vi "solar_tcp Core Client.vi"(7 "Action":T4, 8 "error in (no error)":errorcluster, 9 "Read Timeout (0ms)":i32, 10 "Message to Send":string, 11 "TCP Data in":T1 {"Debug"."Time" format="%<%Y-%m-%d\n%H:%M:%S%3u>T"}) -> (0 "error out":errorcluster, 1 "Connected":bool, 2 "Message Read/Sent":string, 3 "TCP Data out":T1 {"Debug"."Time" format="%<%Y-%m-%d\n%H:%M:%S%3u>T"})   [LabVIEW 2018]
doc: "This is the TCP Client core state machine that handles a TCP session. The <b>Message to Send</b> and <b>Message Read</b> should contain the entire TCP message including the header. Before writing the <b>Message to Send</b> the length field is updated as defined by the configuration header length offset and size. The total length field is typically the first 4 bytes of the message which includes the total packet size."
uses:
  solar_tcp_ctl Action.ctl
  solar_tcp_ctl Data.ctl
  solar_tcp_ctl Config.ctl
  solar_tcp_ctl Debug.ctl
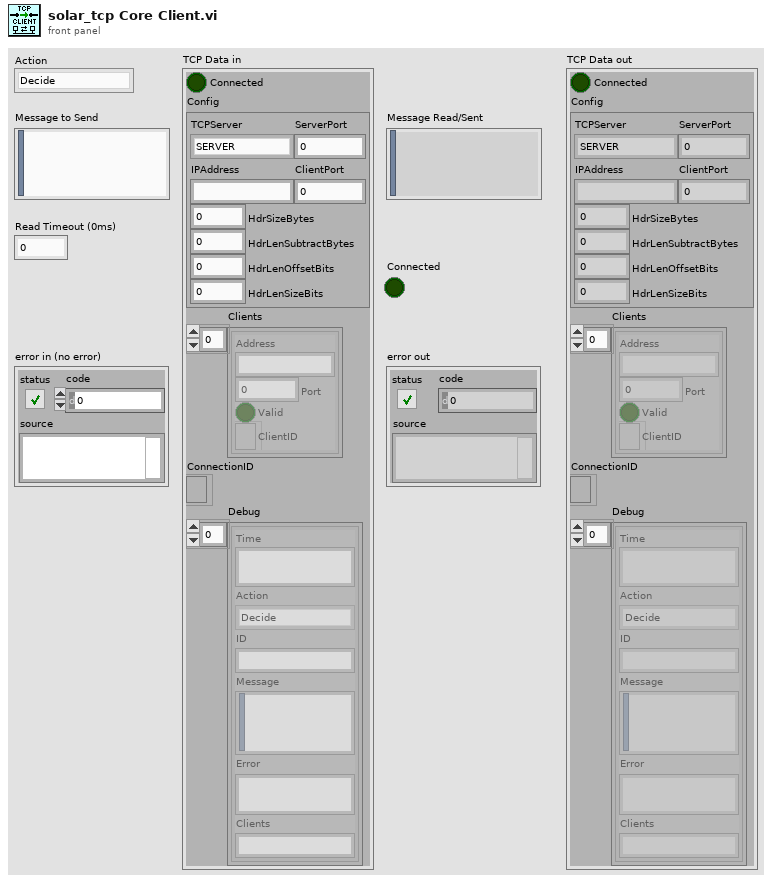
[diagram p1: front panel]
types:
  T1 = typedef "solar_tcp_ctl Data.ctl" = cluster{"Connected":bool, "Config":T2, "Clients":cluster{"Address":string, "Port":u16, "Valid":bool, "ClientID":refnum<k5>}[], "ConnectionID":refnum<k5>, "Debug":T3[]}
  T2 = typedef "solar_tcp_ctl Config.ctl" = cluster{"TCPServer":enum8{"SERVER", "CLIENT"}, "ServerPort":u16, "IPAddress":string, "ClientPort":u16, "HdrSizeBytes":i32, "HdrLenSubtractBytes":i32, "HdrLenOffsetBits":i32, "HdrLenSizeBits":i32}
  T3 = typedef "solar_tcp_ctl Debug.ctl" = cluster{"Time":timestamp, "Action":T4, "ID":string, "Message":string, "Error":string, "Clients":string}
  T4 = typedef "solar_tcp_ctl Action.ctl" = enum16{"Decide", "CreateListener", "Open", "Read", "Write", "Close", "Shutdown", "Done", "ChangePort"}
  T5 = cluster{"Address":string, "Port":u16, "Valid":bool, "ClientID":refnum<k5>}[]
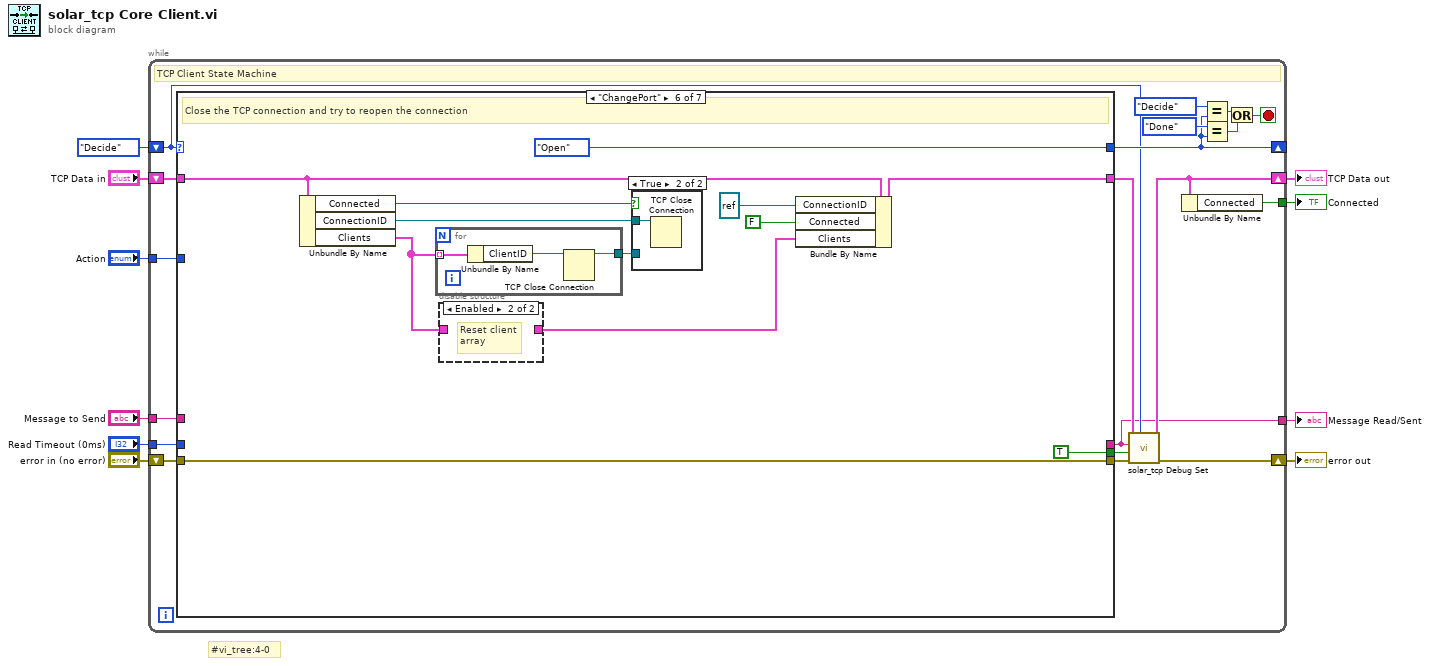
[diagram p0: block diagram]
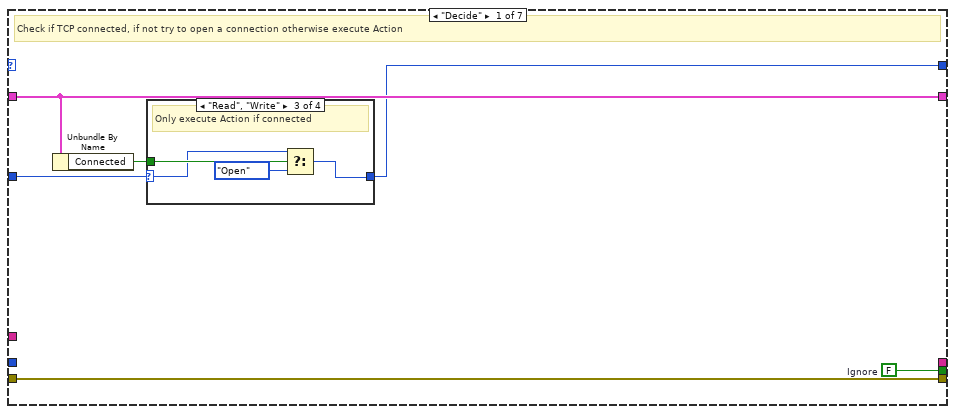
[diagram p2: hidden frame]
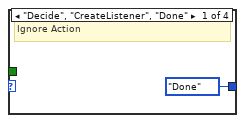
[diagram p3: hidden frame]
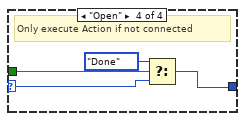
[diagram p5: hidden frame]
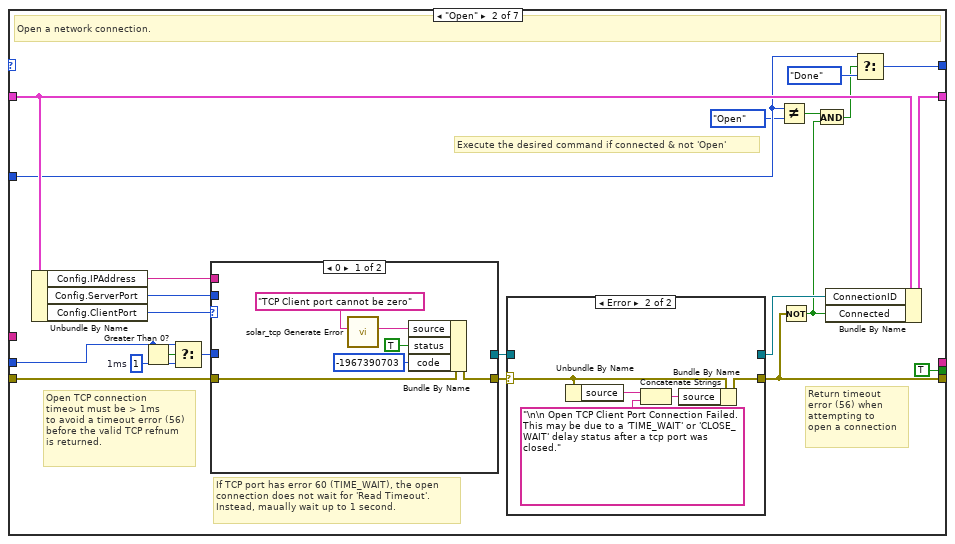
[diagram p6: hidden frame]
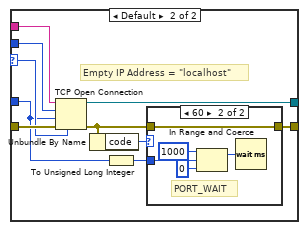
[diagram p7: hidden frame]
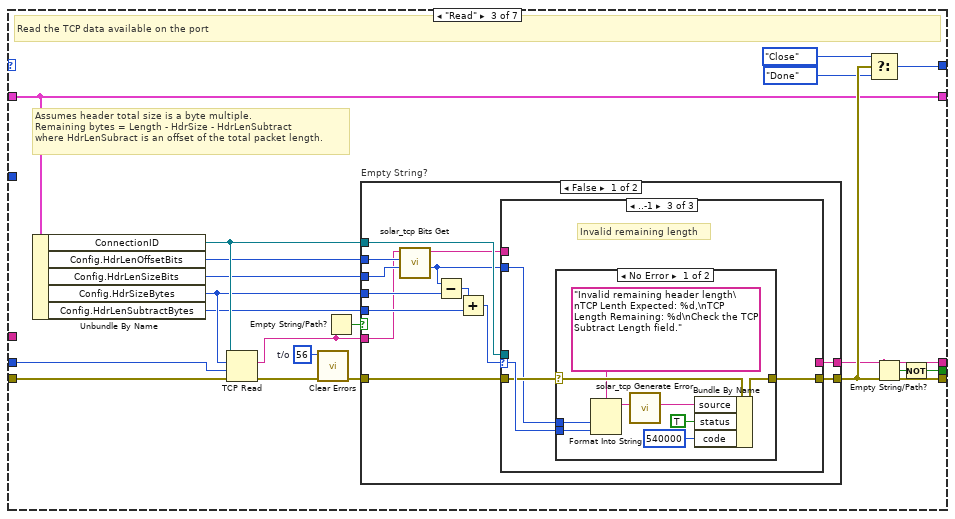
[diagram p10: hidden frame]
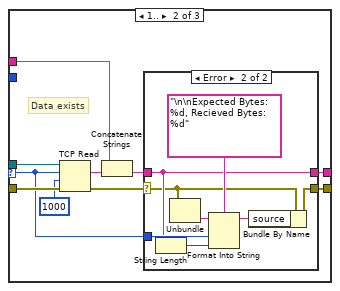
[diagram p12: hidden frame]
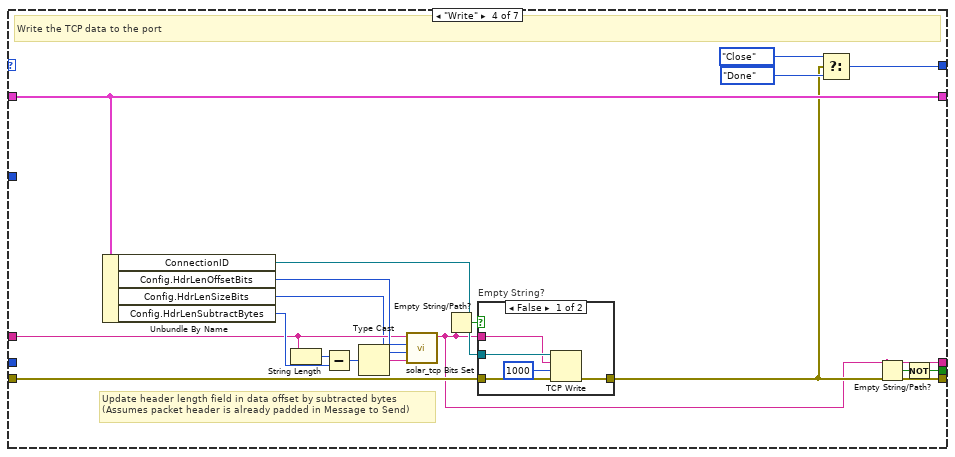
[diagram p16: hidden frame]
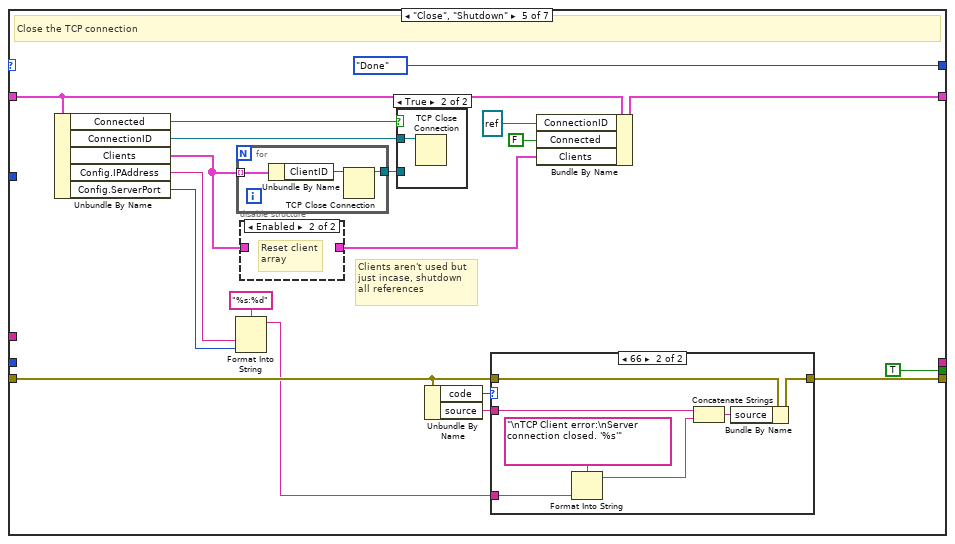
[diagram p18: hidden frame]
diagram:
  # "#vi_tree:4-0"
  n1 = while {
    shift-right: [w18] -> _
    shift-left: solar_tcp_ctl_Action."Decide" ("Function 2") -> [w13]
    shift-right: [w15] -> w5
    shift-left: "TCP Data in" -> [w29]
    tunnel: [w12] -> w10
    tunnel: "Action" -> [w25]
    tunnel: "Message to Send" -> [w22]
    shift-right: [w17] -> w2
    shift-left: "error in (no error)" -> [w21]
    tunnel: "Read Timeout (0ms)" -> [w20]
    tunnel: [w19] -> w1
    stop <- w26 stop-if-true
    # "TCP Client State Machine"
    n2 = case shown="\"ChangePort\"" w13 {
      tunnel: w29 -> [w35 w67 w110 w182 w202 w226 w244]
      tunnel: [w35 w66 w110 w182 w201 w225 w244] -> w14
      tunnel: [w33 w58 w116 w185 solar_tcp_ctl_Action."Done" ("Action 2") solar_tcp_ctl_Action."Open" ("Action 2") solar_tcp_ctl_Action."Done" ("Function 2")] -> w18
      tunnel: [w31 w46 w114 w181 w196 w234 w242] -> w16
      tunnel: [_ _ w99 w170 _ _ _] -> w12
      tunnel: w25 -> [w32 w56 _ _ _ _ _]
      tunnel: w22 -> [_ _ _ w175 _ _ _]
      tunnel: w21 -> [w31 w60 w111 w179 w197 w234 w242]
      tunnel: w20 -> [_ w48 w103 _ _ _ _]
      tunnel: [w30 TRUE ("Ignore") w97 w168 TRUE TRUE w241] -> w11
      frame "Decide" {
        w30 = FALSE  # Ignore
        # "Check if TCP connected, if not try to open a connection otherwise execute Action"
        n3 = Unbundle By Name(w35) -> ("Connected"=w34:bool)
        n4 = case shown="\"Read\", \"Write\"" w32 {
          selector: w32 -> [_ w37 w39 w43]
          tunnel: w34 -> [_ _ w41 w45]
          tunnel: [solar_tcp_ctl_Action."Done" ("Action 2") w37 w40 w44] -> w33
          frame "Decide", "CreateListener", "Done" {
            # "Ignore Action"
          }
          frame "Close", "Shutdown", "ChangePort" {
            # "Always Execute Action"
          }
          frame "Read", "Write" {
            # "Only execute Action if connected"
            n5 = Select(t=w39, s=w41, f=solar_tcp_ctl_Action."Open" ("Action 2")) -> (s? t:f=w40:T4)
          }
          frame "Open" {
            # "Only execute Action if not connected"
            n6 = Select(t=solar_tcp_ctl_Action."Done", s=w45, f=w43) -> (s? t:f=w44:T4)
          }
        }
      }
      frame "Open" {
        w50 = 1  # 1ms
        # "Return timeout\nerror (56) when\nattempting to\nopen a connection"
        # "Open TCP connection\ntimeout must be > 1ms\nto avoid a timeout error (56)\nbefore the valid TCP refnum\nis returned."
        # "If TCP port has error 60 (TIME_WAIT), the open\nconnection does not wait for 'Read Timeout'.\nInstead, maually wait up to 1 second."
        # "Execute the desired command if connected & not 'Open'"
        # "Open a network connection."
        n7 = Unbundle By Name(w67) -> ("Config.IPAddress"=w63:string, "Config.ServerPort"=w64:u16, "Config.ClientPort"=w59:u16)
        n8 = Greater Than 0?(x=w48) -> (x > 0?=w49:bool)
        n9 = Select(t=w48, s=w49, f=w50) -> (s? t:f=w47:i32)
        n10 = case shown="0" w59 {
          selector: w59 -> [_ w79]
          tunnel: [w72 w76] -> w65
          tunnel: w64 -> [_ w83]
          tunnel: w63 -> [_ w80]
          tunnel: [_ w82] -> w62
          tunnel: w60 -> [w73 w81]
          tunnel: w47 -> [_ w74]
          frame 0 {
            n11 = call "solar_tcp Generate Error.vi"("Source in"="TCP Client port cannot be zero" ("source")) -> ("Source + Call Chain"=w71:string)  [unwired: 10 in]
            n12 = Bundle By Name(cluster=w73, "source"=w71, "status"=TRUE, "code"=-1967390703 ("error code (0)")) -> (w72:errorcluster)
          }
          frame Default {
            # "Empty IP Address = \"localhost\""
            n13 = TCP Open Connection(address=w80, remote port or service name=w83, timeout ms (60000)=w74, local port=w79, error in (no error)=w81) -> (connection ID=w82:refnum<k5>, error out=w75:errorcluster)
            n14 = Unbundle By Name(w75) -> ("code"=w77:i32)
            n15 = To Unsigned Long Integer(number=w74) -> (unsigned 32bit integer=w78:u32)
            n16 = case shown="60" w77 {
              tunnel: w78 -> [_ w86]
              tunnel: [w84 w85] -> w76
              tunnel: w75 -> [w84 w85]
              frame Default {
              }
              frame 60 {
                # "PORT_WAIT"
                n17 = In Range and Coerce(upper limit=u32 1000, x=w86, lower limit=u32 0 ("f")) -> (coerced(x)=w87:u32)  [unwired: 1 out]
                n18 = Wait (ms)(milliseconds to wait=w87) -> ()  [unwired: 1 out]
              }
            }
          }
        }
        n19 = case shown="Error" w65 {
          selector: w65 -> [w91 w95]
          tunnel: [w91 w96] -> w46
          tunnel: w62 -> [w90 _]
          tunnel: [w90 _] -> w61
          frame No Error {
          }
          frame Error {
            n20 = Unbundle By Name(w95) -> ("source"=w93:string)
            n21 = Concatenate Strings(w93, "\n\n Open TCP Client Port Connection Failed. This may be due to a 'TIME_WAIT' or 'CLOSE_WAIT' delay status after a tcp port was closed.") -> (w94:string)
            n22 = Bundle By Name(cluster=w95, "source"=w94) -> (w96:errorcluster)
          }
        }
        n23 = Not Equal?(x=w56, y=solar_tcp_ctl_Action."Open" ("x")) -> (x != y?=w55:bool)
        n24 = Not(x=w46) -> (.not. x?=w52:bool)
        n25 = And(x=w55, y=w52) -> (x .and. y?=w54:bool)
        n26 = Bundle By Name(cluster=w67, "ConnectionID"=w61, "Connected"=w52) -> (w66:T1)
        n27 = Select(t=w56, s=w54, f=solar_tcp_ctl_Action."Done" ("Action")) -> (s? t:f=w58:T4)
      }
      frame "Read" {
        w102 = 56  # t/o
        # "Assumes header total size is a byte multiple. \nRemaining bytes = Length - HdrSize - HdrLenSubtract\nwhere HdrLenSubract is an offset of the total packet length."
        # "Read the TCP data available on the port"
        n28 = Unbundle By Name(w110) -> ("ConnectionID"=w115:refnum<k5>, "Config.HdrLenOffsetBits"=w109:i32, "Config.HdrLenSizeBits"=w108:i32, "Config.HdrSizeBytes"=w107:i32, "Config.HdrLenSubtractBytes"=w106:i32)
        n29 = TCP Read(connection ID=w115, bytes to read=w107, error in (no error)=w111, 9:w103) -> (data out=w105:string, error out=w101:errorcluster)  [unwired: 1 in, 1 out]
        n30 = call <vilib>:"Clear Errors.vi"("error in (no error)"=w101, "specific error code to clear (0: all)"=w102) -> ("error out"=w100:errorcluster)  [unwired: 4 in, 1 out]
        n31 = Empty String/Path?(string/path=w105) -> (empty?=w104:bool)
        n32 = case "Empty String?" shown="False" w104 {
          tunnel: w115 -> [w129 _]
          tunnel: [w128 w167] -> w114
          tunnel: [w127 w166] -> w99
          tunnel: w100 -> [w126 w167]
          tunnel: w109 -> [w125 _]
          tunnel: w108 -> [w124 _]
          tunnel: w107 -> [w123 _]
          tunnel: w106 -> [w121 _]
          tunnel: w105 -> [w120 w166]
          frame False {
            n33 = call "solar_tcp Bits Get.vi"("Bit Size (0..64)"=w124, "Bit Offset (0)"=w125, "Data"=w120) -> ("Value as I32"=w117:i32, "dup Data"=w118:string)  [unwired: 6 in, 1 out]
            n34 = Subtract(x=w117, y=w123) -> (x-y=w122:i32)
            n35 = Add(x=w122, y=w121) -> (x+y=w119:i32)
            n36 = case shown="..-1" w119 {
              selector: w119 -> [_ w135 w154]
              tunnel: w129 -> [_ w141 _]
              tunnel: [w130 w140 w155] -> w128
              tunnel: [w131 w139 _] -> w127
              tunnel: w126 -> [w130 w138 w153]
              tunnel: w118 -> [w131 w132 _]
              tunnel: w117 -> [_ _ w152]
              frame 0 {
                # "No more data expected\n- Return tcp data"
              }
              frame 1.. {
                # "Data exists"
                n37 = TCP Read(connection ID=w141, bytes to read=w135, error in (no error)=w138, 9:1000 ("Timeout (ms)")) -> (data out=w136:string, error out=w137:errorcluster)  [unwired: 1 in, 1 out]
                n38 = Concatenate Strings(w132, w136) -> (w133:string)
                n39 = case shown="Error" w137 {
                  selector: w137 -> [w143 w145]
                  tunnel: w133 -> [w142 w146]
                  tunnel: w135 -> [_ w149]
                  tunnel: [w143 w148] -> w140
                  tunnel: [w142 w146] -> w139
                  frame No Error {
                    # "Return entire message\n(including header)"
                  }
                  frame Error {
                    n40 = String Length(string=w146) -> (length=w151:i32)
                    n41 = Unbundle(w145) -> ("source"=w144:string)  [unwired: 2 out]
                    n42 = Format Into String(format string="\n\nExpected Bytes: %d, Recieved Bytes: %d" ("source"), initial string=w144, w149, w151) -> (resulting string=w147:string)  [unwired: 1 in, 1 out]
                    n43 = Bundle By Name(cluster=w145, "source"=w147) -> (w148:errorcluster)
                  }
                }
              }
              frame ..-1 {
                # "Invalid remaining length"
                n44 = case shown="No Error" w153 {
                  selector: w153 -> [w163 w165]
                  tunnel: w154 -> [w160 _]
                  tunnel: [w164 w165] -> w155
                  tunnel: w152 -> [w159 _]
                  frame No Error {
                    n45 = Format Into String(format string="Invalid remaining header length\nTCP Lenth Expected: %d,\nTCP Length Remaining: %d\nCheck the TCP Subtract Length field." ("source"), w159, w160) -> (resulting string=w157:string)  [unwired: 2 in, 1 out]
                    n46 = call "solar_tcp Generate Error.vi"("Source in"=w157) -> ("Source + Call Chain"=w156:string)  [unwired: 10 in]
                    n47 = Bundle By Name(cluster=w163, "source"=w156, "status"=TRUE, "code"=540000) -> (w164:errorcluster)
                  }
                  frame Error {
                  }
                }
              }
            }
          }
          frame True {
          }
        }
        n48 = Select(t=solar_tcp_ctl_Action."Close" ("Action 2"), s=w114, f=solar_tcp_ctl_Action."Done" ("Action 2")) -> (s? t:f=w116:T4)
        n49 = Empty String/Path?(string/path=w99) -> (empty?=w98:bool)
        n50 = Not(x=w98) -> (.not. x?=w97:bool)
      }
      frame "Write" {
        # "Update header length field in data offset by subtracted bytes\n(Assumes packet header is already padded in Message to Send)"
        # "Write the TCP data to the port"
        n51 = Unbundle By Name(w182) -> ("ConnectionID"=w180:refnum<k5>, "Config.HdrLenOffsetBits"=w176:i32, "Config.HdrLenSizeBits"=w173:i32, "Config.HdrLenSubtractBytes"=w177:i32)
        n52 = String Length(string=w175) -> (length=w178:i32)
        n53 = Subtract(x=w178, y=w177) -> (x-y=w172:i32)
        n54 = Type Cast(x=w172) -> (*(type *) &x=w171:string)  [unwired: 1 in]
        n55 = call "solar_tcp Bits Set.vi"("Value (Binary) [Byte Aligned]"=w171, "Bit Size (0..64)"=w173, "Bit Offset (0)"=w176, "Buffered Data in"=w175) -> ("Data out"=w170:string)  [unwired: 7 in]
        n56 = Empty String/Path?(string/path=w170) -> (empty?=w174:bool)
        n57 = case "Empty String?" shown="False" w174 {
          tunnel: w179 -> [w189 w191]
          tunnel: [w188 w191] -> w181
          tunnel: w180 -> [w187 _]
          tunnel: w170 -> [w186 _]
          frame False {
            n58 = TCP Write(connection ID=w187, data in=w186, error in (no error)=w189, 9:1000 ("timeout ms (25000)")) -> (error out=w188:errorcluster)  [unwired: 2 out]
          }
          frame True {
          }
        }
        n59 = Select(t=solar_tcp_ctl_Action."Close" ("Action 2"), s=w181, f=solar_tcp_ctl_Action."Done" ("Action 2")) -> (s? t:f=w185:T4)
        n60 = Empty String/Path?(string/path=w170) -> (empty?=w169:bool)
        n61 = Not(x=w169) -> (.not. x?=w168:bool)
      }
      frame "Close", "Shutdown" {
        # "Clients aren't used but\njust incase, shutdown\nall references"
        # "Close the TCP connection"
        n62 = Unbundle By Name(w202) -> ("Connected"=w207:bool, "ConnectionID"=w206:refnum<k5>, "Clients"=w203:T5, "Config.IPAddress"=w195:string, "Config.ServerPort"=w194:u16)
        n63 = Format Into String(format string="%s:%d", w195, w194) -> (resulting string=w192:string)  [unwired: 2 in, 1 out]
        n64 = for {
          tunnel: w203 -> [w222] mode=indexing
          tunnel: [w220] -> w205
          n65 = Unbundle By Name(w222) -> ("ClientID"=w221:refnum<k5>)
          n66 = TCP Close Connection(connection ID=w221) -> (connection ID out=w220:refnum<k5>)  [unwired: 2 in, 1 out]
        }
        n67 = disable-structure shown="Enabled" {
          disable-tunnel: [w219 _] -> w204
          disable-tunnel: w203 -> [w219 _]
          frame Disabled {
          }
          frame Enabled {
            # "Reset client\narray"
          }
        }
        n68 = case shown="True" w207 {
          tunnel: w206 -> [_ w223]
          tunnel: w205 -> [_ _]
          frame False {
          }
          frame True {
            n69 = TCP Close Connection(connection ID=w223) -> ()  [unwired: 2 in, 2 out]
          }
        }
        n70 = Unbundle By Name(w197) -> ("code"=w199:i32, "source"=w198:string)
        n71 = case shown="66" w199 {
          tunnel: [w211 w217] -> w196
          tunnel: w197 -> [w211 w218]
          tunnel: w198 -> [_ w216]
          tunnel: w192 -> [_ w212]
          frame Default {
          }
          frame 66 {
            n72 = Format Into String(format string="\nTCP Client error:\nServer connection closed. '%s'", w212) -> (resulting string=w213:string)  [unwired: 2 in, 1 out]
            n73 = Concatenate Strings(w216, w213) -> (w215:string)
            n74 = Bundle By Name(cluster=w218, "source"=w215) -> (w217:errorcluster)
          }
        }
        n75 = Bundle By Name(cluster=w202, "ConnectionID"=refnum<k5> refnum ("Connection ID"), "Connected"=FALSE, "Clients"=w204) -> (w201:T1)
      }
      frame "ChangePort" {
        # "Close the TCP connection and try to reopen the connection"
        n76 = Unbundle By Name(w226) -> ("Connected"=w231:bool, "ConnectionID"=w230:refnum<k5>, "Clients"=w227:T5)
        n77 = for {
          tunnel: w227 -> [w239] mode=indexing
          tunnel: [w237] -> w229
          n78 = Unbundle By Name(w239) -> ("ClientID"=w238:refnum<k5>)
          n79 = TCP Close Connection(connection ID=w238) -> (connection ID out=w237:refnum<k5>)  [unwired: 2 in, 1 out]
        }
        n80 = disable-structure shown="Enabled" {
          disable-tunnel: [w236 _] -> w228
          disable-tunnel: w227 -> [w236 _]
          frame Disabled {
          }
          frame Enabled {
            # "Reset client\narray"
          }
        }
        n81 = case shown="True" w231 {
          tunnel: w230 -> [_ w240]
          tunnel: w229 -> [_ _]
          frame False {
          }
          frame True {
            n82 = TCP Close Connection(connection ID=w240) -> ()  [unwired: 2 in, 2 out]
          }
        }
        n83 = Bundle By Name(cluster=w226, "ConnectionID"=refnum<k5> refnum ("Connection ID"), "Connected"=FALSE, "Clients"=w228) -> (w225:T1)
      }
      frame "CreateListener", "Done" {
        w241 = FALSE  # Ignore
        # "Do Nothing"
      }
    }
    n84 = call "solar_tcp Debug Set.vi"("Action"=w13, "error in (no error)"=w16, "Update? (T)"=w11, "Message Sent/Read"=w12, "TCP Data in"=w14) -> ("error out"=w17:errorcluster, "TCP Data out"=w15:T1)  [unwired: 5 in]
    n85 = Unbundle By Name(w15) -> ("Connected"=w19:bool)
    n86 = Equal?(x=solar_tcp_ctl_Action."Decide" ("Action 2"), y=w18) -> (x = y?=w28:bool)
    n87 = Equal?(x=solar_tcp_ctl_Action."Done" ("Action 2"), y=w18) -> (x = y?=w27:bool)
    n88 = Or(x=w28, y=w27) -> (x .or. y?=w26:bool)
  }
  "error out" <- w2
  "Message Read/Sent" <- w10
  "TCP Data out" <- w5
  "Connected" <- w1
